vi "GetTranslatorCount.vi"() -> (4 "Number Of Translations":i32)   [LabVIEW 2011]
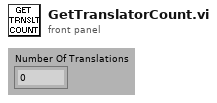
[diagram p1: front panel]
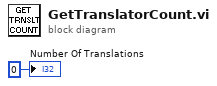
[diagram p0: block diagram]
diagram:
  "Number Of Translations" <- 0 ("Number Of Translations")
